vi "BRig_dataTrial_sSelection.vi"() -> (2 "output_sSelection":i32)   [LabVIEW 2014]
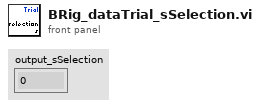
[diagram p1: front panel]
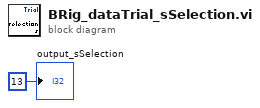
[diagram p0: block diagram]
diagram:
  "output_sSelection" <- 13 ("output_iBlock")
